vi "prop_action_buttons.vi"() -> ()   [LabVIEW 2020, in "3DPC_SurfacePlot.xctl"]
uses:
  <vilib>/Native 3D Graph/xcontrol/3DPC_SurfacePlot.xctl
  <vilib>/Utility/miscctls.llb/LVPointTypeDef.ctl
panel:
  in  "tab":i16
  out "commit":bool=TRUE
  in  "Help Button":bool
  in  "Cancel Button":bool
  in  "quit":refnum<user-event>
  in  "Ok Button":bool
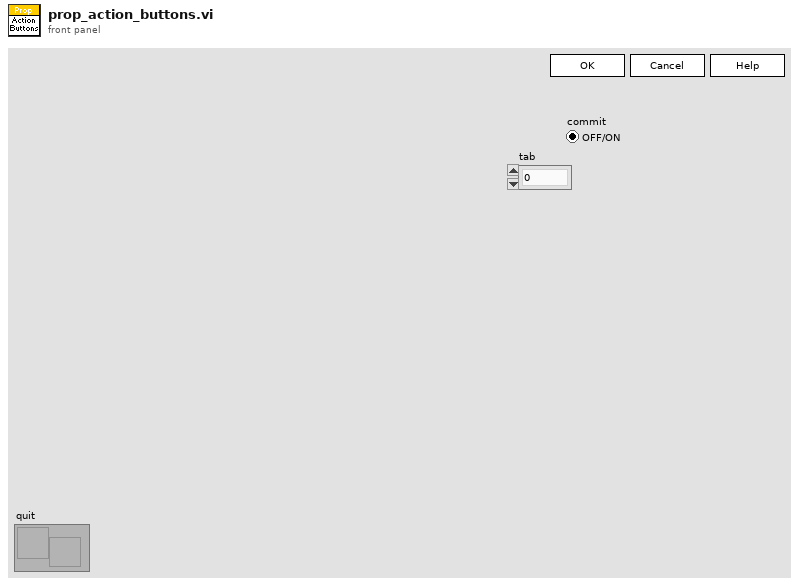
[diagram p1: front panel]
types:
  T1 = typedef "LVPointTypeDef.ctl" = cluster{"Horizontal":i16, "Vertical":i16}
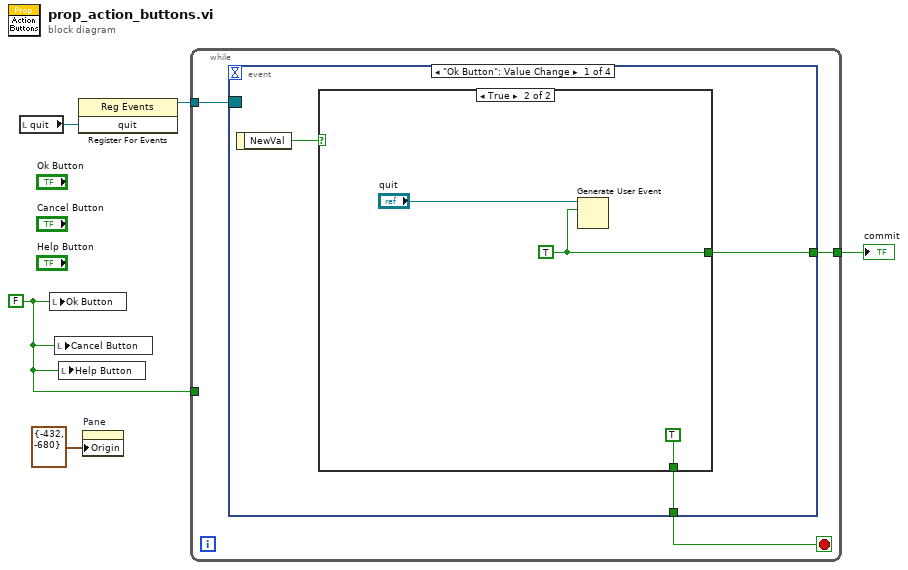
[diagram p0: block diagram]
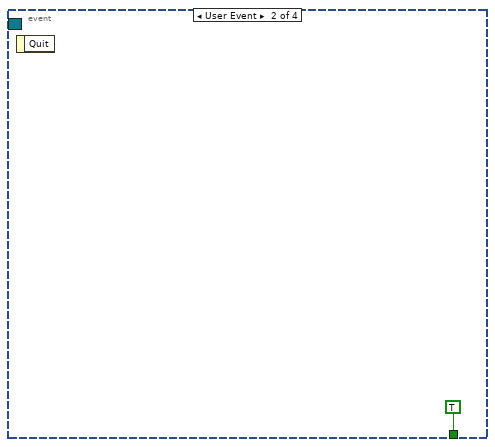
[diagram p3: hidden frame]
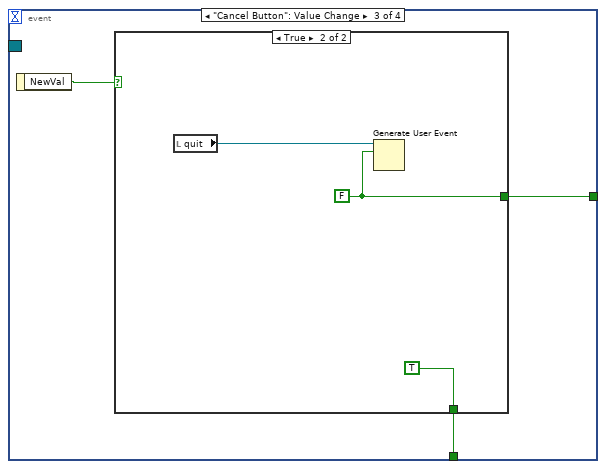
[diagram p4: hidden frame]
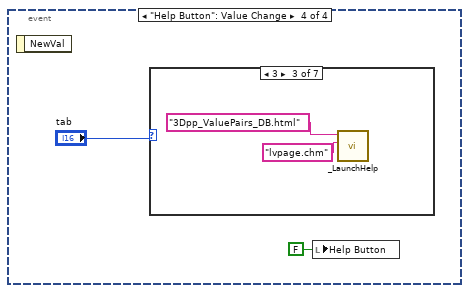
[diagram p6: hidden frame]
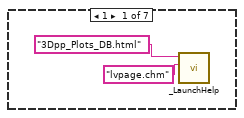
[diagram p7: hidden frame]
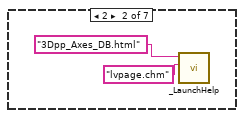
[diagram p8: hidden frame]
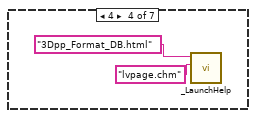
[diagram p9: hidden frame]
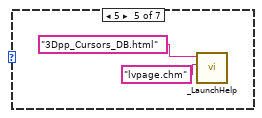
[diagram p10: hidden frame]
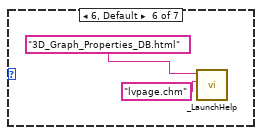
[diagram p11: hidden frame]
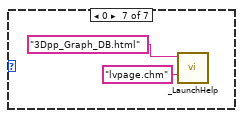
[diagram p12: hidden frame]
diagram:
  w3 = FALSE ("Ok Button")
  n1 = local read "quit"() -> (w2:refnum<user-event>)
  n2 = local write "Ok Button"(w3) -> ()
  n3 = local write "Cancel Button"(w3) -> ()
  n4 = local write "Help Button"(w3) -> ()
  n5 = register-events(w2) -> (reference out=w1:refnum<event-registration>)  [unwired: 2 in, 1 out]
  n6 = property on="Pane" class="Pane"("Origin"=T1 {"Horizontal"=-432, "Vertical"=-680} ("Point")) -> ()  [unwired: 2 in, 2 out]
  n7 = while {
    tunnel: [w8] -> w5
    tunnel: w3 -> [_]
    tunnel: w1 -> [w6]
    stop <- w7 stop-if-true
    n8 = event shown="[0] \"Ok Button\": Value Change" {
      selector: w6 -> [_ _ _ _]
      dyn-events: _ -> [_ _ _ _]
      timeout: _ -> [_ _ _ _]
      tunnel: [w10 _ w17 _] -> w8
      tunnel: [w9 TRUE ("event data") w16 _] -> w7
      event "Ok Button": Value Change {
        n9 = event-data() -> ("NewVal"=w11:bool)  [unwired: 1 out]
        n10 = case shown="True" w11 {
          tunnel: [_ w13] -> w10
          tunnel: [_ TRUE ("event data")] -> w9
          frame False {
          }
          frame True {
            w13 = TRUE ("event data")
            n11 = Generate User Event(user event="quit", event data cluster=w13) -> ()  [unwired: 2 in, 2 out]
          }
        }
      }
      event User Event {
        n12 = event-data() -> ()  [unwired: 2 out]
      }
      event "Cancel Button": Value Change {
        n13 = event-data() -> ("NewVal"=w18:bool)  [unwired: 1 out]
        n14 = case shown="True" w18 {
          tunnel: [_ w20] -> w17
          tunnel: [_ TRUE ("event data")] -> w16
          frame False {
          }
          frame True {
            w20 = FALSE ("event data")
            n15 = local read "quit"() -> (w21:refnum<user-event>)
            n16 = Generate User Event(user event=w21, event data cluster=w20) -> ()  [unwired: 2 in, 2 out]
          }
        }
      }
      event "Help Button": Value Change {
        n17 = event-data() -> ()  [unwired: 2 out]
        n18 = case shown="3" "tab" {
          frame 1 {
            n19 = call <helpdir>:"_LaunchHelp.vi"("CHM or HLP filename (lvdialog.chm)"="lvpage.chm", "HTML filename"="3Dpp_Plots_DB.html") -> ()  [unwired: 1 in, 5 out]
          }
          frame 2 {
            n20 = call <helpdir>:"_LaunchHelp.vi"("CHM or HLP filename (lvdialog.chm)"="lvpage.chm", "HTML filename"="3Dpp_Axes_DB.html") -> ()  [unwired: 1 in, 5 out]
          }
          frame 3 {
            n21 = call <helpdir>:"_LaunchHelp.vi"("CHM or HLP filename (lvdialog.chm)"="lvpage.chm", "HTML filename"="3Dpp_ValuePairs_DB.html") -> ()  [unwired: 1 in, 5 out]
          }
          frame 4 {
            n22 = call <helpdir>:"_LaunchHelp.vi"("CHM or HLP filename (lvdialog.chm)"="lvpage.chm", "HTML filename"="3Dpp_Format_DB.html") -> ()  [unwired: 1 in, 5 out]
          }
          frame 5 {
            n23 = call <helpdir>:"_LaunchHelp.vi"("CHM or HLP filename (lvdialog.chm)"="lvpage.chm", "HTML filename"="3Dpp_Cursors_DB.html") -> ()  [unwired: 1 in, 5 out]
          }
          frame 6, Default {
            n24 = call <helpdir>:"_LaunchHelp.vi"("CHM or HLP filename (lvdialog.chm)"="lvpage.chm", "HTML filename"="3D_Graph_Properties_DB.html") -> ()  [unwired: 1 in, 5 out]
          }
          frame 0 {
            n25 = call <helpdir>:"_LaunchHelp.vi"("CHM or HLP filename (lvdialog.chm)"="lvpage.chm", "HTML filename"="3Dpp_Graph_DB.html") -> ()  [unwired: 1 in, 5 out]
          }
        }
        n26 = local write "Help Button"(FALSE ("Help Button")) -> ()
      }
    }
  }
  "commit" <- w5
